vi "VISA_WRITE_READ_SUBVI.vi"(5 "Command":string="*IDN?", 6 "VISA resource name":refnum<visa-resource-name>="COM1", 7 "Read 2":bool, 8 "Write 2":bool) -> (0 "error out":errorcluster, 3 "Response":string)   [LabVIEW 2022 SP3]
panel:
  in  "Read Count":u32=1000
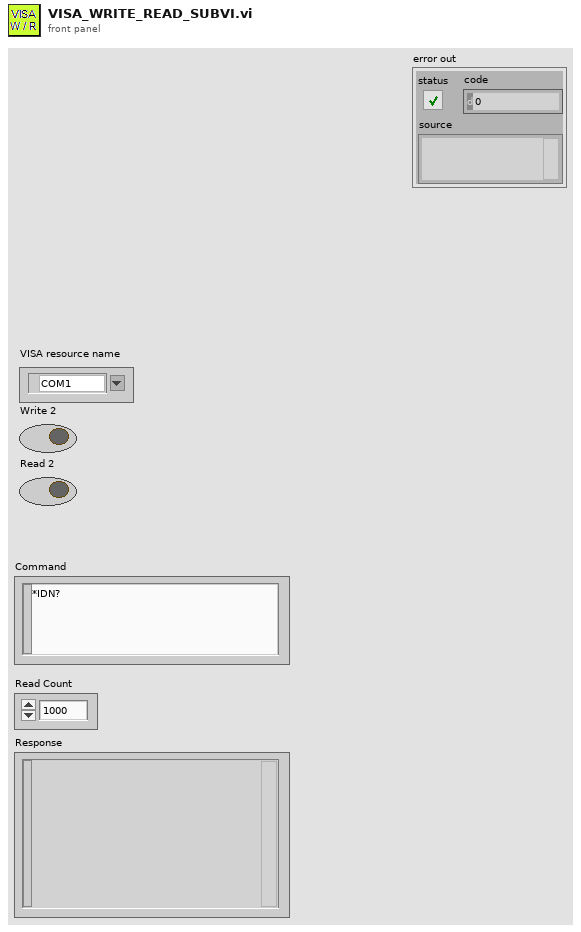
[diagram p1: front panel]
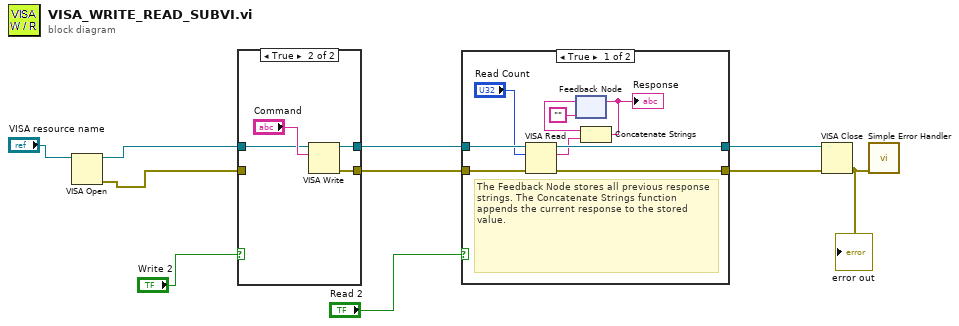
[diagram p0: block diagram]
diagram:
  n1 = VISA Open(VISA resource name="VISA resource name") -> (VISA resource name=w7:refnum<visa-resource-name>, error out=w5:errorcluster)  [unwired: 4 in]
  n2 = case shown="True" "Write 2" {
    tunnel: w7 -> [w12 w15]
    tunnel: [w12 w14] -> w4
    tunnel: [w11 w13] -> w3
    tunnel: w5 -> [w11 _]
    frame False {
    }
    frame True {
      n3 = VISA Write(VISA resource name=w15, write buffer="Command") -> (VISA resource name out=w14:refnum<visa-resource-name>, error out=w13:errorcluster)  [unwired: 1 in, 1 out]
    }
  }
  n4 = case shown="True" "Read 2" {
    tunnel: [w23 w27] -> w8
    tunnel: w4 -> [w25 w27]
    tunnel: [w21 w26] -> w9
    tunnel: w3 -> [w24 w26]
    frame True {
      # "The Feedback Node stores all previous response strings. The Concatenate Strings function appends the current response to the stored value."
      n5 = VISA Read(VISA resource name=w25, byte count="Read Count", error in (no error)=w24) -> (VISA resource name out=w23:refnum<visa-resource-name>, read buffer=w20:string, error out=w21:errorcluster)  [unwired: 1 out]
      n6 = feedback #1("") -> (w19:string)
      n7 = Concatenate Strings(w19, w20) -> (w18:string)
      "Response" <- w18
      n8 = feedback-in #1(w18) -> ()
    }
    frame False {
    }
  }
  n9 = VISA Close(VISA resource name=w8, error in (no error)=w9) -> (error out=w10:errorcluster)
  "error out" <- w10
  n10 = call <vilib>:"Simple Error Handler.vi"("error in (no error)"=w10) -> ()  [unwired: 1 in, 8 out]
